vi "Select Test Configuration.vi"(8 "error in (no error)":errorcluster) -> (0 "error out":errorcluster, 2 "Type":string, 5 "Cancelled?":bool)   [LabVIEW 2015]
panel:
  in  "Cancel Button":bool
  in  "Gas":i32(listbox)
  in  "OK Button":bool
  out "Test Sequence":i32(listbox)=-2
  # "Select Test Configuration"
  # "Please select the type of\ntest you would like to configure."
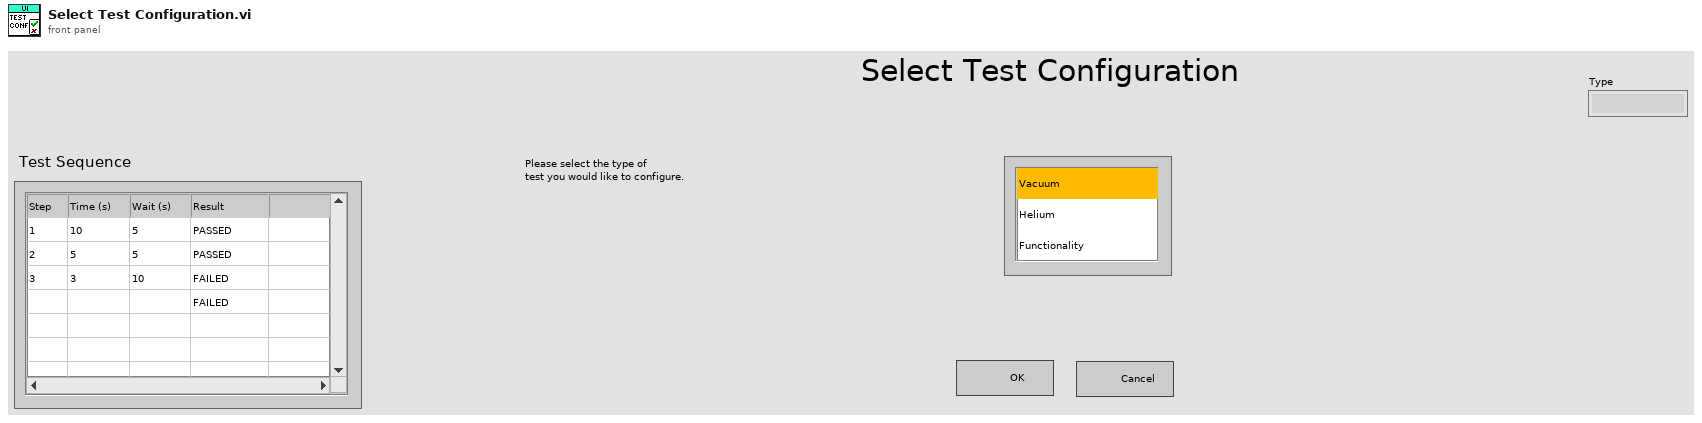
[diagram p1: front panel]
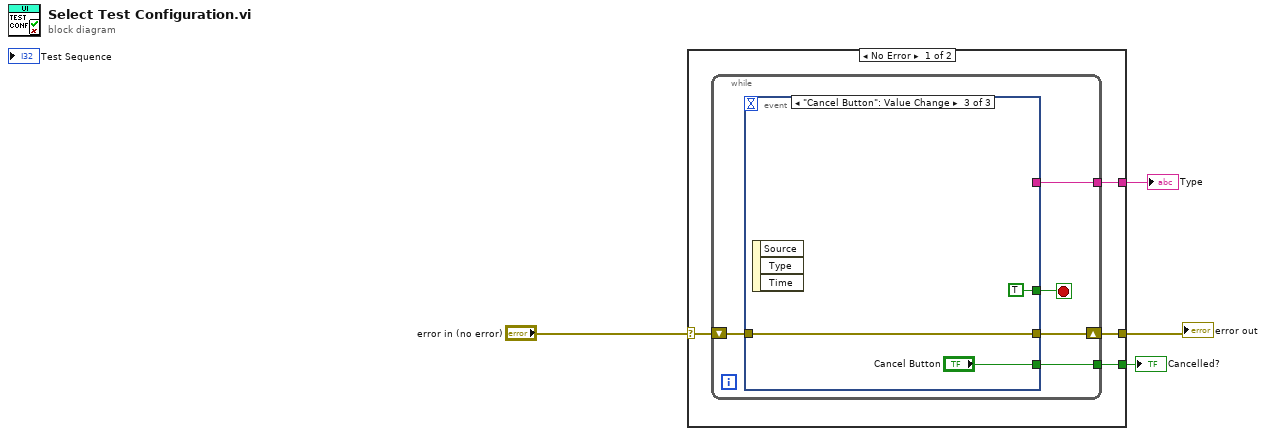
[diagram p0: block diagram]
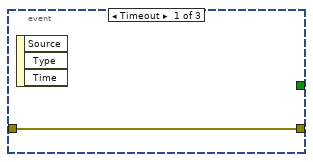
[diagram p2: hidden frame]
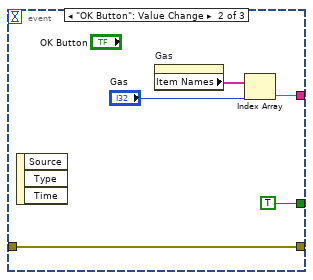
[diagram p3: hidden frame]
diagram:
  n1 = case shown="No Error" "error in (no error)" {
    selector: "error in (no error)" -> [w8 w23]
    tunnel: [w7 w23] -> w4
    tunnel: [w6 _] -> w2
    tunnel: [w5 _] -> w1
    frame No Error {
      n2 = while {
        shift-right: [w10] -> w7
        shift-left: w8 -> [w11]
        tunnel: [w12] -> w6
        tunnel: [w9] -> w5
        stop <- w13 stop-if-true
        n3 = event shown="[2] \"Cancel Button\": Value Change" {
          selector: _ -> [_ _ _]
          dyn-events: _ -> [_ _ _]
          timeout: _ -> [_ _ _]
          tunnel: [_ TRUE TRUE] -> w13
          tunnel: [_ w16 _] -> w12
          tunnel: w11 -> [w14 w15 w22]
          tunnel: [w14 w15 w22] -> w10
          tunnel: [_ _ "Cancel Button"] -> w9
          event Timeout {
            n4 = event-data() -> ()  [unwired: 1 in, 3 out]
          }
          event "OK Button": Value Change {
            n5 = event-data() -> ()  [unwired: 1 in, 3 out]
            n6 = property on="Gas" class="LstBox (strict)"() -> ("Item Names"=w18:string[])  [unwired: 2 in, 2 out]
            n7 = Index Array(array=w18, index="Gas") -> (element=w16:string)
          }
          event "Cancel Button": Value Change {
            n8 = event-data() -> ()  [unwired: 1 in, 3 out]
          }
        }
      }
    }
    frame Error {
    }
  }
  "error out" <- w4
  "Type" <- w2
  "Cancelled?" <- w1
